vi "IterationDurationToDt.vi"(11 "Iteration Duration":i64) -> (3 "Numeric":dbl)   [LabVIEW 2018, in "Pid.lvlib"]
uses:
  Pid.lvlib
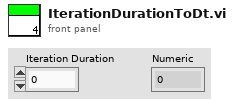
[diagram p1: front panel]
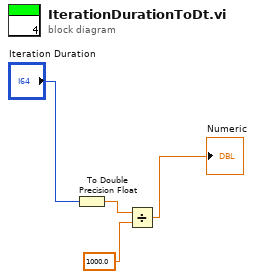
[diagram p0: block diagram]
diagram:
  n1 = To Double Precision Float(number="Iteration Duration") -> (double precision float=w2:dbl)
  n2 = Divide(x=w2, y=1000.0) -> (x/y=→"Numeric":dbl)
